vi "server.vi"(11 "array":i32[][](array[numeric])) -> (0 "error":bool)   [LabVIEW 2022 SP3]
doc: "Creates a named service and listens on the first available port. When a client connects to the service, it sends a response string to the client."
panel:
  in  "stop":bool
  in  "Numeric":dbl
  # "將一8*8陣列轉換為一字串並作為名為2OtheFlooR234的server上傳直到有人接收"
  # "Overview: Demonstrates the use of the TCP functions to initialize a named TCP service that can send data to a client VI.\nInstructions:\n1. Run the VI.\n2. Open TCP Named Service - Client.vi and follow the instructions on its front panel.\n3. Click Stop to stop the VI."
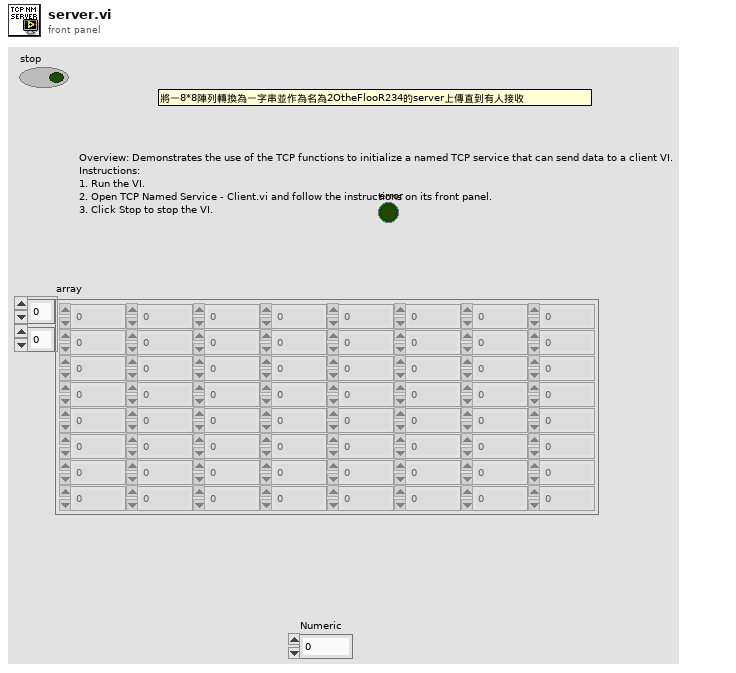
[diagram p1: front panel]
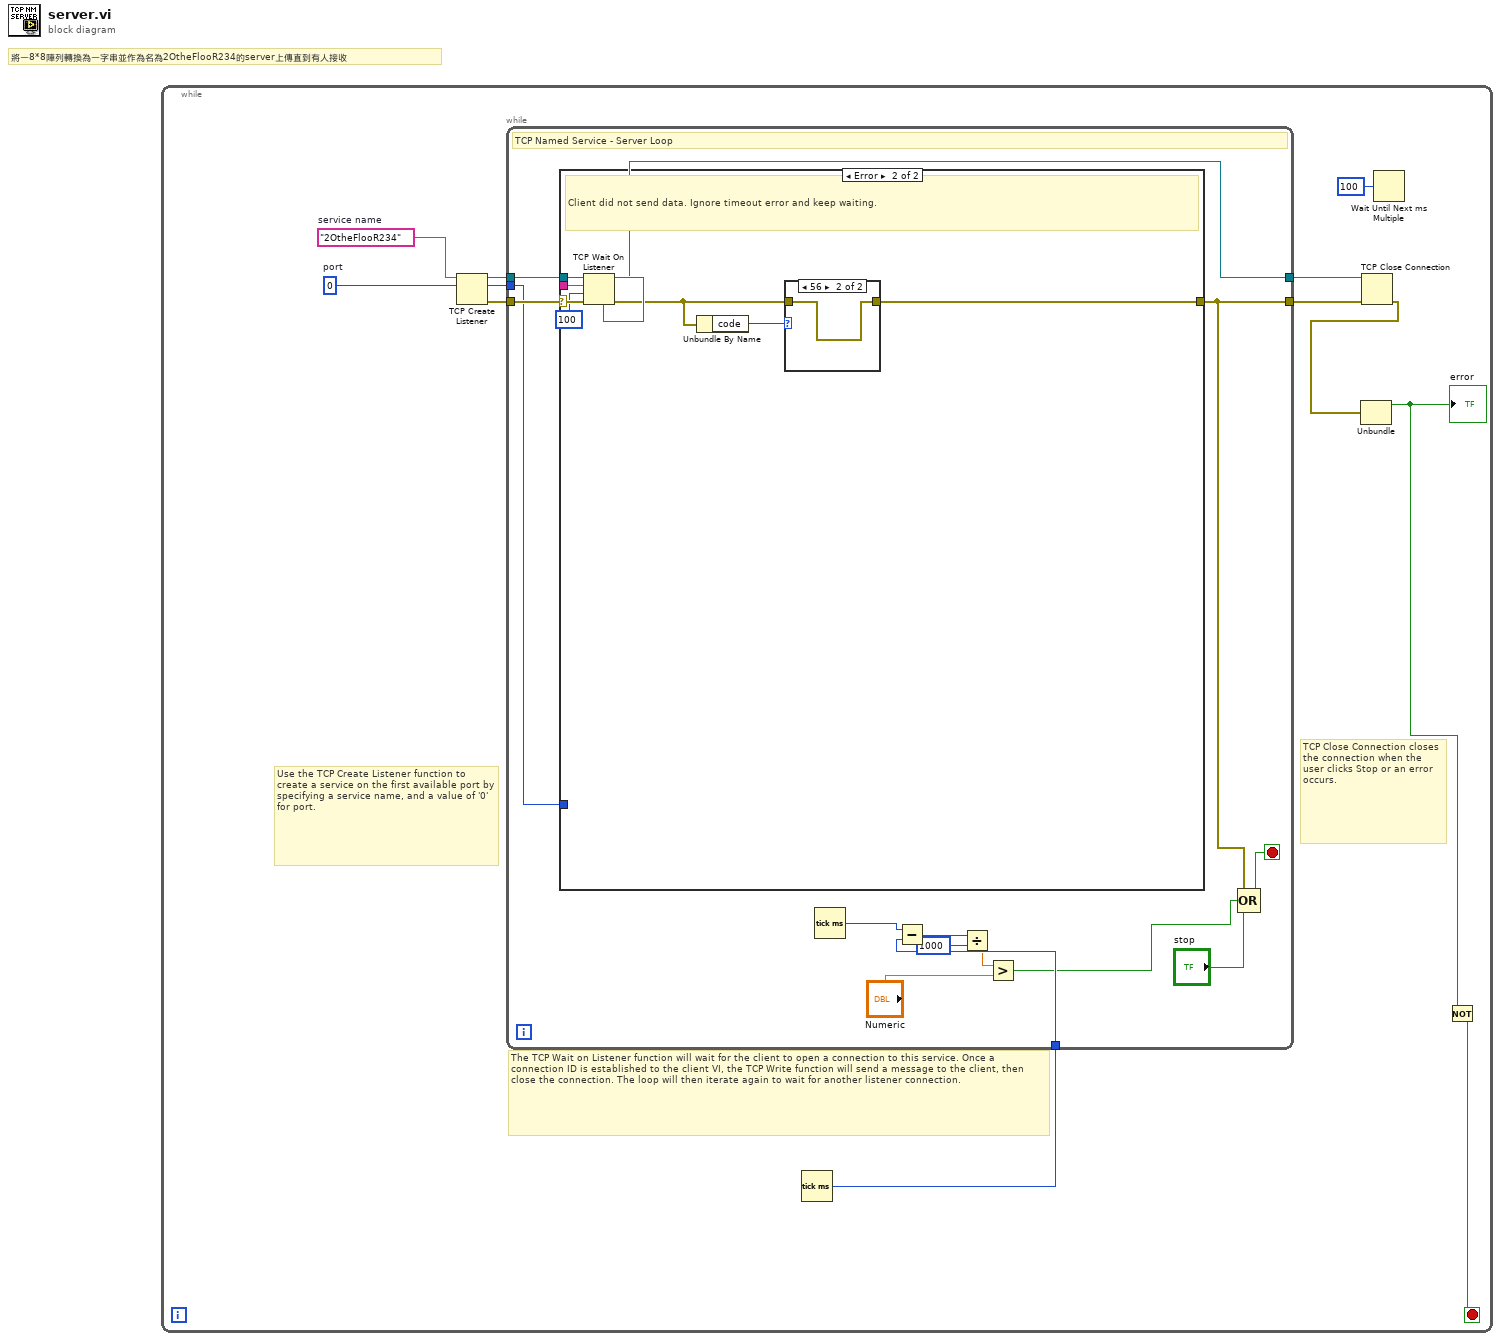
[diagram p0: block diagram]
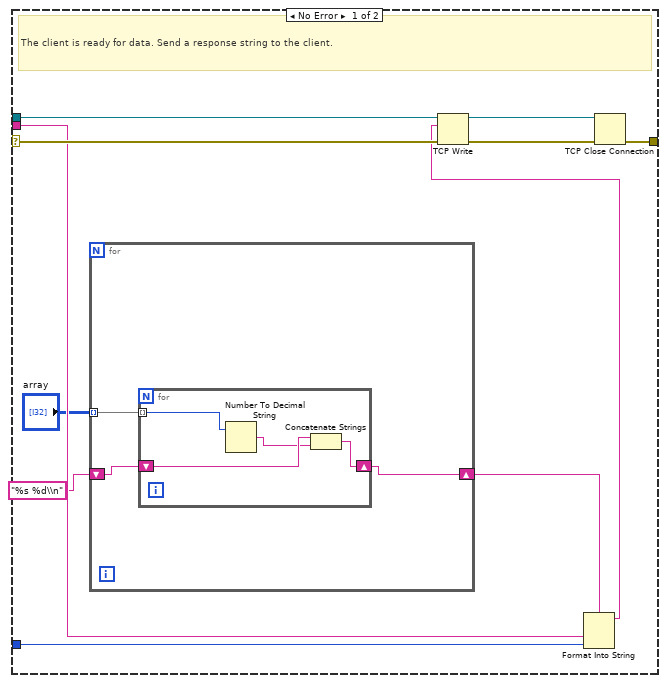
[diagram p2: hidden frame]
diagram:
  # "將一8*8陣列轉換為一字串並作為名為2OtheFlooR234的server上傳直到有人接收"
  n1 = while {
    stop <- w3 stop-if-true
    w8 = u16 0  # port
    w7 = "2OtheFlooR234"  # service name
    # "TCP Close Connection closes the connection when the user clicks Stop or an error occurs."
    # "The TCP Wait on Listener function will wait for the client to open a connection to this service. Once a connection ID is established to the client VI, the TCP Write function will send a message to the client, then close the connection. The loop will then iterate again to wait for another listener connection."
    # "Use the TCP Create Listener function to create a service on the first available port by specifying a service name, and a value of '0' for port."
    n2 = TCP Create Listener(10:w8, 11:w7) -> (0:w11:errorcluster, 2:w9:u16, 3:w12:refnum<k5>)  [unwired: 3 in]
    n3 = Tick Count (ms)() -> (millisecond timer value=w6:u32)
    n4 = while {
      tunnel: [w15] -> w5
      tunnel: w12 -> [w30]
      tunnel: w11 -> [w28]
      tunnel: [w23] -> w10
      tunnel: w9 -> [w26]
      tunnel: w6 -> [w20]
      stop <- w13 stop-if-true
      # "TCP Named Service - Server Loop"
      n5 = TCP Wait On Listener(8:w28, 9:100 ("timeout ms (25000)"), 11:w30) -> (0:w29:errorcluster, 2:w24:string, 3:w23:refnum<k5>, 4:w27:refnum<k5>)  [unwired: 1 in, 1 out]
      n6 = case shown="Error" w29 {
        selector: w29 -> [w41 w51]
        tunnel: [w35 w49] -> w15
        tunnel: w27 -> [w36 _]
        tunnel: w26 -> [w39 _]
        tunnel: w24 -> [w38 _]
        frame No Error {
          # "The client is ready for data. Send a response string to the client."
          n7 = for {
            shift-right: [w43] -> w33
            shift-left: "%s %d\\n" -> [w44]
            tunnel: "array" -> [w42] mode=indexing
            n8 = for {
              shift-right: [w46] -> w43
              shift-left: w44 -> [w48]
              tunnel: w42 -> [w45] mode=indexing
              n9 = Number To Decimal String(number=w45) -> (decimal integer string=w47:string)  [unwired: 1 in]
              n10 = Concatenate Strings(w48, w47) -> (w46:string)
            }
          }
          n11 = Format Into String(format string=w33, w38, w39) -> (resulting string=w37:string)  [unwired: 2 in, 1 out]
          n12 = TCP Write(connection ID=w36, data in=w37, error in (no error)=w41) -> (connection ID out=w34:refnum<k5>, error out=w40:errorcluster)  [unwired: 1 in, 1 out]
          n13 = TCP Close Connection(connection ID=w34, error in (no error)=w40) -> (error out=w35:errorcluster)  [unwired: 1 in, 1 out]
        }
        frame Error {
          # "Client did not send data. Ignore timeout error and keep waiting."
          n14 = Unbundle By Name(w51) -> ("code"=w50:i32)
          n15 = case shown="56" w50 {
            tunnel: w51 -> [w52 w53]
            tunnel: [w52 w53] -> w49
            frame Default {
            }
            frame 56 {
            }
          }
        }
      }
      n16 = Tick Count (ms)() -> (millisecond timer value=w21:u32)
      n17 = Subtract(x=w21, y=w20) -> (x-y=w19:u32)
      n18 = Divide(x=w19, y=u32 1000) -> (x/y=w17:dbl)
      n19 = Greater?(x=w17, y="Numeric") -> (0:w16:bool)
      n20 = Compound Arithmetic op=OR(w15, w16, "stop") -> (w13:bool)
    }
    n21 = TCP Close Connection(connection ID=w10, error in (no error)=w5) -> (error out=w2:errorcluster)  [unwired: 1 in, 1 out]
    n22 = Unbundle(w2) -> ("status"=w4:bool)  [unwired: 2 out]
    "error" <- w4
    n23 = Wait Until Next ms Multiple(millisecond multiple=u32 100) -> ()  [unwired: 1 out]
    n24 = Not(x=w4) -> (.not. x?=w3:bool)
  }
